vi "Create File.vi"(8 "Start Path":path, 9 "Default File Name":string, 11 "File Extension":string="*.bmp") -> (1 "canceled?":bool=TRUE, 3 "File Path":path)   [LabVIEW 2018]
panel:
  out "error out":errorcluster
  # "Output"
  # "Inputs"
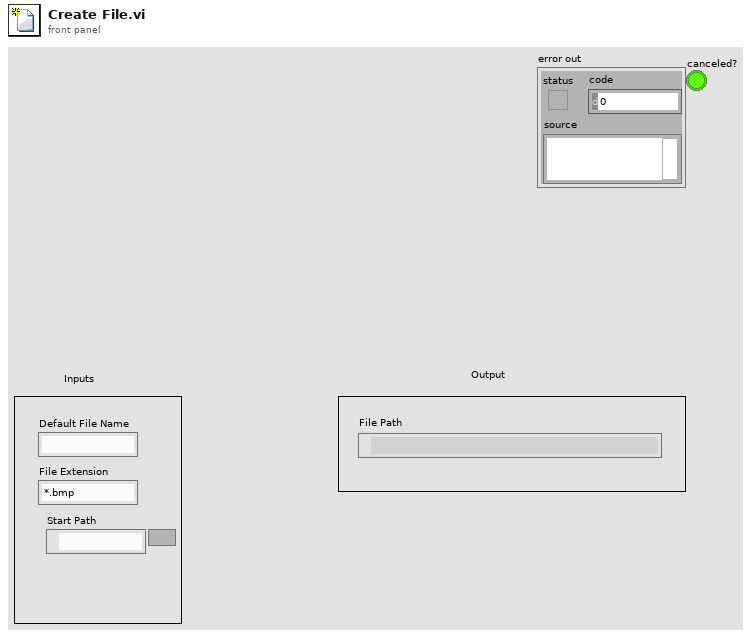
[diagram p1: front panel]
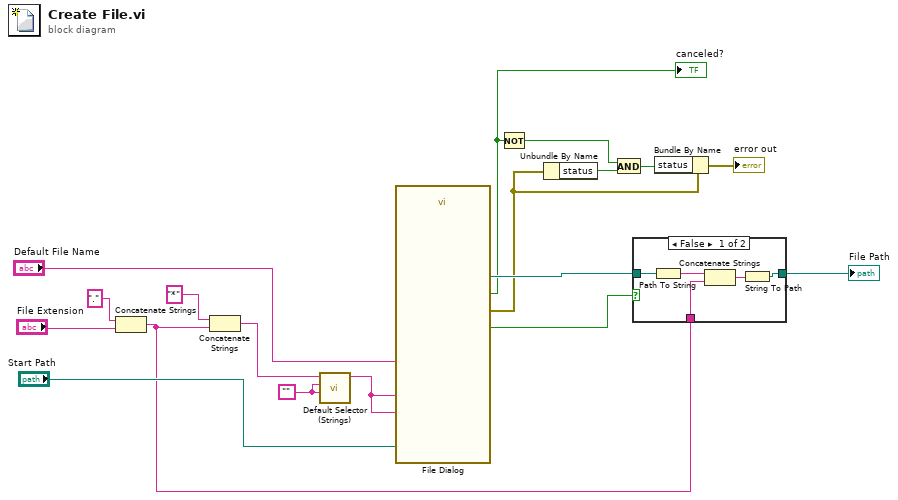
[diagram p0: block diagram]
diagram:
  w18 = ""
  n1 = Concatenate Strings(".", "File Extension") -> (w9:string)
  n2 = Concatenate Strings("*", w9) -> (w10:string)
  n3 = call "Default Selector (Strings).vi"("Null String"=w18, "Default Sting"=w18, "Input String"=w10) -> ("Output String"=w13:string)  [unwired: 8 in]
  n4 = call "File Dialog"("start path"="Start Path", "default name"="Default File Name", "pattern (all files)"=w13, "pattern label"=w13) -> ("selected path"=w17:path, "exists"=w16:bool, "cancelled"=w1:bool, "error out"=w4:errorcluster)  [unwired: 8 in]
  "canceled?" <- w1
  n5 = Not(x=w1) -> (.not. x?=w5:bool)
  n6 = Unbundle By Name(w4) -> ("status"=w6:bool)
  n7 = And(x=w5, y=w6) -> (x .and. y?=w3:bool)
  n8 = case shown="False" w16 {
    tunnel: w17 -> [w22 w24]
    tunnel: [w21 w24] -> w14
    tunnel: w9 -> [w19 _]
    frame False {
      n9 = Path To String(path=w22) -> (string=w23:string)
      n10 = Concatenate Strings(w23, w19) -> (w20:string)
      n11 = String To Path(string=w20) -> (path=w21:path)
    }
    frame True {
    }
  }
  "File Path" <- w14
  n12 = Bundle By Name(cluster=w4, "status"=w3) -> (→"error out":errorcluster)
